vi "_free.vi"(9 "error in (no error)":errorcluster, 10 "MDPtr DVR":refnum<data-value>) -> (2 "error out":errorcluster)   [LabVIEW 2017, in "MDPtr.lvlib"]
uses:
  MDPtr.lvlib
  MDPtr TypeDef/MDPtr DataFrame-Memory.ctl
  MDPtr TypeDef/MDPtr DataFrame-Common.ctl
  <vilib>/Utility/Data Type/Type Definitions/Data Type.ctl
  Error Handler/_Build Error Cluster.vi
  <vilib>/Utility/Data Type/NI_Data Type.lvlib
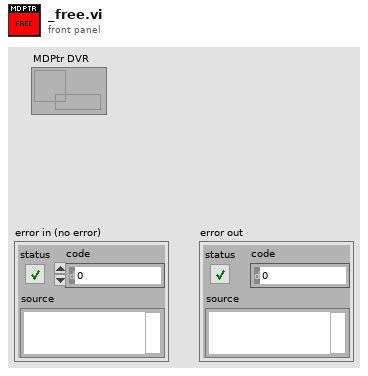
[diagram p1: front panel]
types:
  T1 = typedef "MDPtr.lvlib/MDPtr DataFrame-Memory.ctl" = cluster{"Common":T2, "DVR":refnum<data-value>}
  T2 = typedef "MDPtr.lvlib/MDPtr DataFrame-Common.ctl" = cluster{"Data Type":T3, "Copy Count":i32, "String Attribute":string, "Cache Length":i32, "Data Length":i32}
  T3 = typedef "NI_Data Type.lvlib/Data Type.ctl" = enum8{"Invalid Type", "Void", "I8", "I16", "I32", "I64", "U8", "U16", "U32", "U64", "Single Float", "Double Float", "Extended Float", "Single Complex", "Double Complex", "Extended Complex", "Enum U8", "Enum U16", "Enum U32", "Enum U64", "Single Float With Unit", "Double Float With Unit", "Extended Float With Unit", "Single Complex with Unit", "Double Complex with Unit", "Extended Complex with Unit", "Boolean", "String", "Path", "Picture", "Tag", "Array", "Cluster", "Variant", "LV Variant", "Waveform", "Timestamp", "Digital Waveform", "Digital Data", "ExpressData", "Refnum", "External Data", "VI", "Poly VI", "LabVIEW Class Instance", "Fixed Point"}
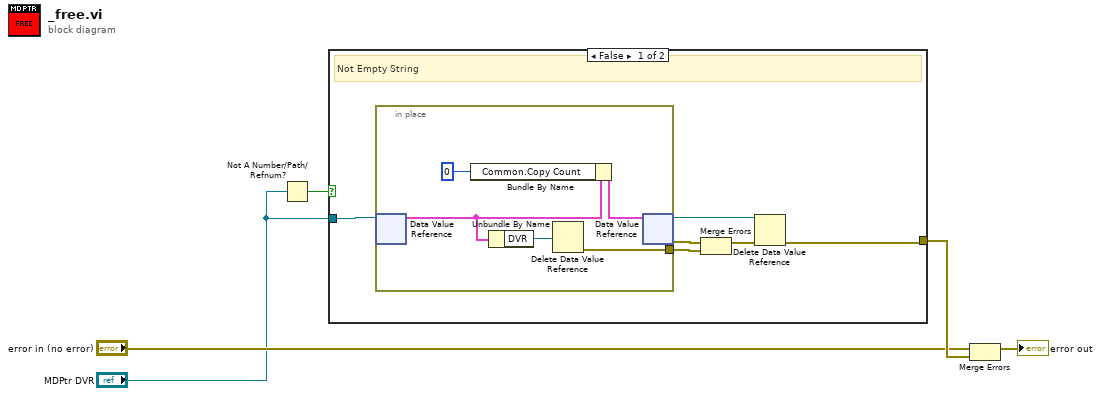
[diagram p0: block diagram]
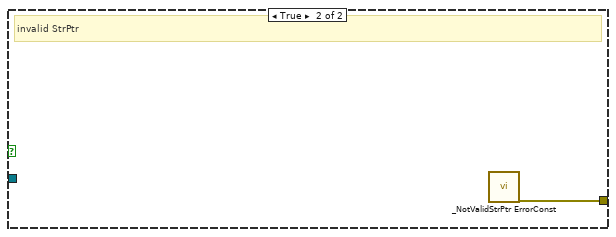
[diagram p2: hidden frame]
diagram:
  n1 = Not A Number/Path/Refnum?(number/path/refnum="MDPtr DVR") -> (NaN/Path/Refnum?=w1:bool)
  n2 = case shown="False" w1 {
    tunnel: [w9 w17] -> w5
    tunnel: "MDPtr DVR" -> [w10 _]
    frame False {
      # "Not Empty String"
      n3 = in-place {
        in-place-border: [w12] -> w6
        n4 = in-place-dvr #1(w10) -> (w16:T1)  [unwired: 1 out]
        n5 = Bundle By Name(cluster=w16, "Common.Copy Count"=0) -> (w15:T1)
        n6 = Unbundle By Name(w16) -> ("DVR"=w13:refnum<data-value>)
        n7 = Delete Data Value Reference(data value reference=w13) -> (error out=w12:errorcluster)  [unwired: 1 in, 1 out]
        n8 = in-place-dvr #1(w15) -> (w8:refnum<data-value>, w11:errorcluster)
      }
      n9 = Merge Errors(w11, w6) -> (w7:errorcluster)
      n10 = Delete Data Value Reference(data value reference=w8, error in=w7) -> (error out=w9:errorcluster)  [unwired: 1 out]
    }
    frame True {
      # "invalid StrPtr"
      n11 = call "_NotValidStrPtr ErrorConst.vi"() -> ("error out"=w17:errorcluster)  [unwired: 19 in]
    }
  }
  n12 = Merge Errors("error in (no error)", w5) -> (→"error out":errorcluster)
